vi "2-4.vi"() -> ()   [LabVIEW 2017]
panel:
  out "数值":dbl
  in  "k":dbl
  in  "x":dbl
  in  "b":dbl
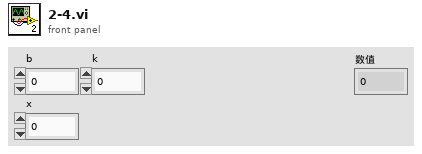
[diagram p1: front panel]
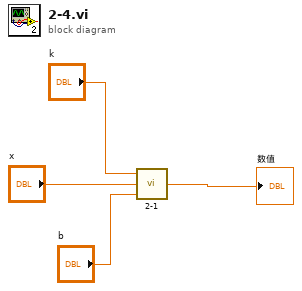
[diagram p0: block diagram]
diagram:
  n1 = call "2-1.vi"("b"="b", "x"="x", "k"="k") -> ("数值"=→"数值":dbl)
